vi "ReadStatus.vi"(0 "object in":refnum<class "CetoniPump.lvclass">, 2 "index":i32, 5 "error in (no error)":errorcluster) -> (14 "object out":refnum<class "CetoniPump.lvclass">, 16 "Fill Level":dbl, 17 "Is pumping":bool, 18 "Actual Flow Rate":dbl, 19 "error out":errorcluster)   [LabVIEW 2021, in "CetoniPump.lvclass"]
uses:
  CetoniPump.lvclass
  CetoniPump.lvclass/CetoniPump.ctl
  Users/olaja/AppData/Local/CETONI_SDK/lib/labview/labbCAN_Pump_API/labbCAN_Pump_API.lvlib
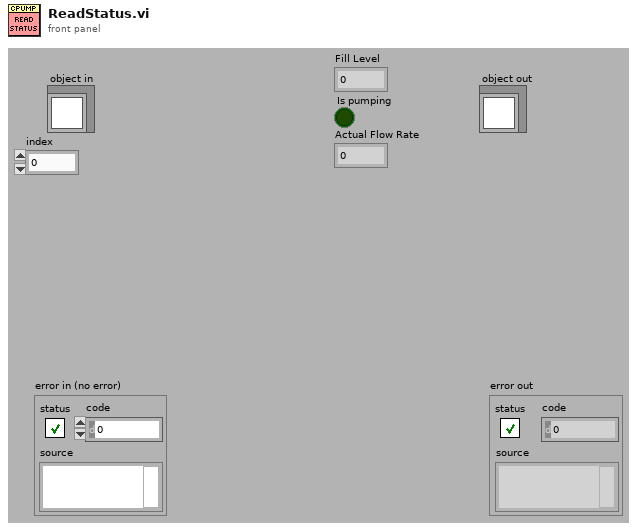
[diagram p1: front panel]
types:
  T1 = cluster{"Pump Handle":i64, "Pump Name":string, "Maximum Volume":dbl, "Maximum Flow Rate":dbl, "Flow Rate":dbl, "Target Level":dbl}[]
  T2 = cluster{"Pump Handle":i64, "Pump Name":string, "Maximum Volume":dbl, "Maximum Flow Rate":dbl, "Flow Rate":dbl, "Target Level":dbl}
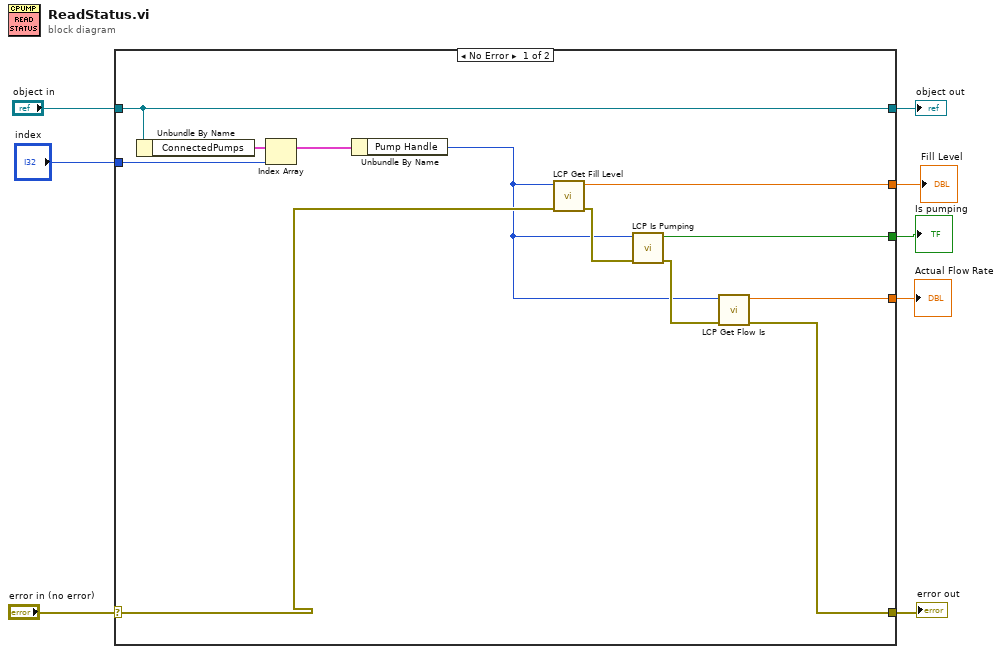
[diagram p0: block diagram]
diagram:
  n1 = case shown="No Error" "error in (no error)" {
    selector: "error in (no error)" -> [w16 w22]
    tunnel: [w15 w22] -> w7
    tunnel: [w20 w21] -> w5
    tunnel: "object in" -> [w20 w21]
    tunnel: [w19 _] -> w4
    tunnel: [w18 _] -> w3
    tunnel: [w14 _] -> w2
    tunnel: "index" -> [w9 _]
    frame No Error {
      n2 = Unbundle By Name(w20) -> ("ConnectedPumps"=w17:T1)
      n3 = Index Array(array=w17, index=w9) -> (element=w10:T2)
      n4 = Unbundle By Name(w10) -> ("Pump Handle"=w11:i64)
      n5 = call "LCP Get Fill Level.vi"("error in (no error)"=w16, "Pump Handle"=w11) -> ("error out"=w13:errorcluster, "Fill Level"=w19:dbl)  [unwired: 8 in]
      n6 = call "LCP Is Pumping.vi"("error in (no error)"=w13, "Pump Handle"=w11) -> ("error out"=w12:errorcluster, "Is pumping"=w18:bool)  [unwired: 8 in]
      n7 = call "LCP Get Flow Is.vi"("error in (no error)"=w12, "Pump Handle"=w11) -> ("error out"=w15:errorcluster, "Actual Flow Rate"=w14:dbl)  [unwired: 8 in]
    }
    frame Error {
    }
  }
  "error out" <- w7
  "object out" <- w5
  "Fill Level" <- w4
  "Is pumping" <- w3
  "Actual Flow Rate" <- w2
